vi "Create from URI String.vi"(10 "error in (no error)":errorcluster, 11 "URI String":string) -> (2 "error out":errorcluster, 3 "URI out":refnum<class "URI.lvclass">)   [LabVIEW 2020, in "Stream.lvlib" / "URI.lvclass"]
uses:
  URI.lvclass
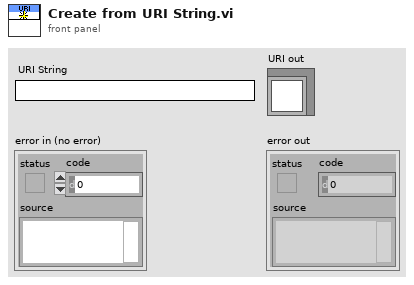
[diagram p1: front panel]
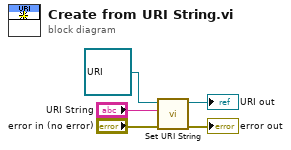
[diagram p0: block diagram]
diagram:
  n1 = call "Set URI String.vi"("error in (no error)"="error in (no error)", "URI String"="URI String", "URI in"=refnum<class "URI.lvclass"> refnum) -> ("error out"=→"error out":errorcluster, "URI out"=→"URI out":refnum<class "URI.lvclass">)  [unwired: 7 in]
